vi "Temperature.vi"() -> ()   [LabVIEW 2018, in "Temperature.lvlib"]
uses:
  Temperature.lvlib
  Modbus.xctl
  Sensor.xctl
  Loop Control.xctl
  General Status.xctl
  <vilib>/Platform/TimedLoop/XDataNode/timing_clust.ctl
  <vilib>/Platform/TimedLoop/XDataNode/nitl_modes.ctl
  <vilib>/Platform/TimedLoop/XDataNode/wakeup.ctl
  <vilib>/platform/TimedLoop/XDataNode/XDataNode.xnode
  <vilib>/Platform/TimedLoop/XDataNode/XDNodeRunTimeDep.lvlib
panel:
  out "General Status":u16(xcontrol)
  in  "Loop Control":T1(xcontrol)
  out "Second":cluster{"Value":sgl, "Medium":sgl, "Status":u16}(xcontrol)
  out "Main":cluster{"Value":sgl, "Medium":sgl, "Status":u16}(xcontrol)
  in  "Modbus":T2(xcontrol)
  out "Chart":sgl[](graph)
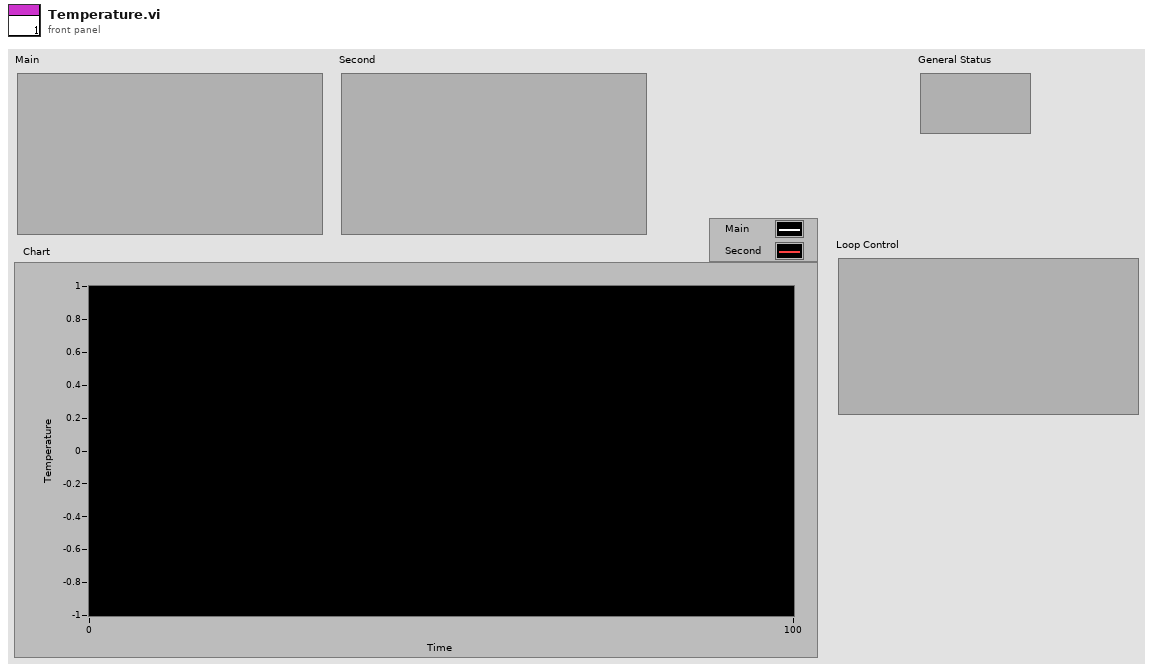
[diagram p1: front panel]
types:
  T1 = cluster{"dt":i64, "error to show":errorcluster, "Active":bool, "stop":bool}
  T2 = cluster{"Communication Error":bool, "Updating":bool, "Off Hook":bool, "Update rate":dbl}
  T3 = typedef "XDNodeRunTimeDep.lvlib/timing_clust.ctl" = cluster{"Expected End [f-1]":u64, "Actual End [f-1]":u64, "Finished Late? [f-1]":bool, "Expected End [i-1]":u64, "Actual End [i-1]":u64, "Finished Late? [i-1]":bool, "Expected Start [i]":u64, "Actual Start [i]":u64, "Expected Start [f]":u64, "Actual Start [f]":u64, "Source Name":string, "Structure Name":string, "Period":i64, "Deadline":i64, "Offset":i64, "Start":i64, "Priority":i32, "Timeout":i32, "Mode":T4, "Wakeup Reason":T5, "Error":errorcluster, "Source Type":string, "Secondary Source Type":string, "Global End Time":u64, "Global Start Time":u64, "Frame Duration":u64, "Iteration Duration":u64, "Assigned CPU":i32, "I/O Scan Engine Mode":u32}
  T4 = typedef "XDNodeRunTimeDep.lvlib/nitl_modes.ctl" = enum32{"No Change", "Process missed periods, maintain original phase", "Discard missed periods, maintain original phase", "Process missed periods, ignore original phase", "Discard missed periods, ignore original phase"}
  T5 = typedef "XDNodeRunTimeDep.lvlib/wakeup.ctl" = enum32{"Normal", "Aborted", "Asynchronous wakeup", "Timing source error", "Timed loop error", "Timeout"}
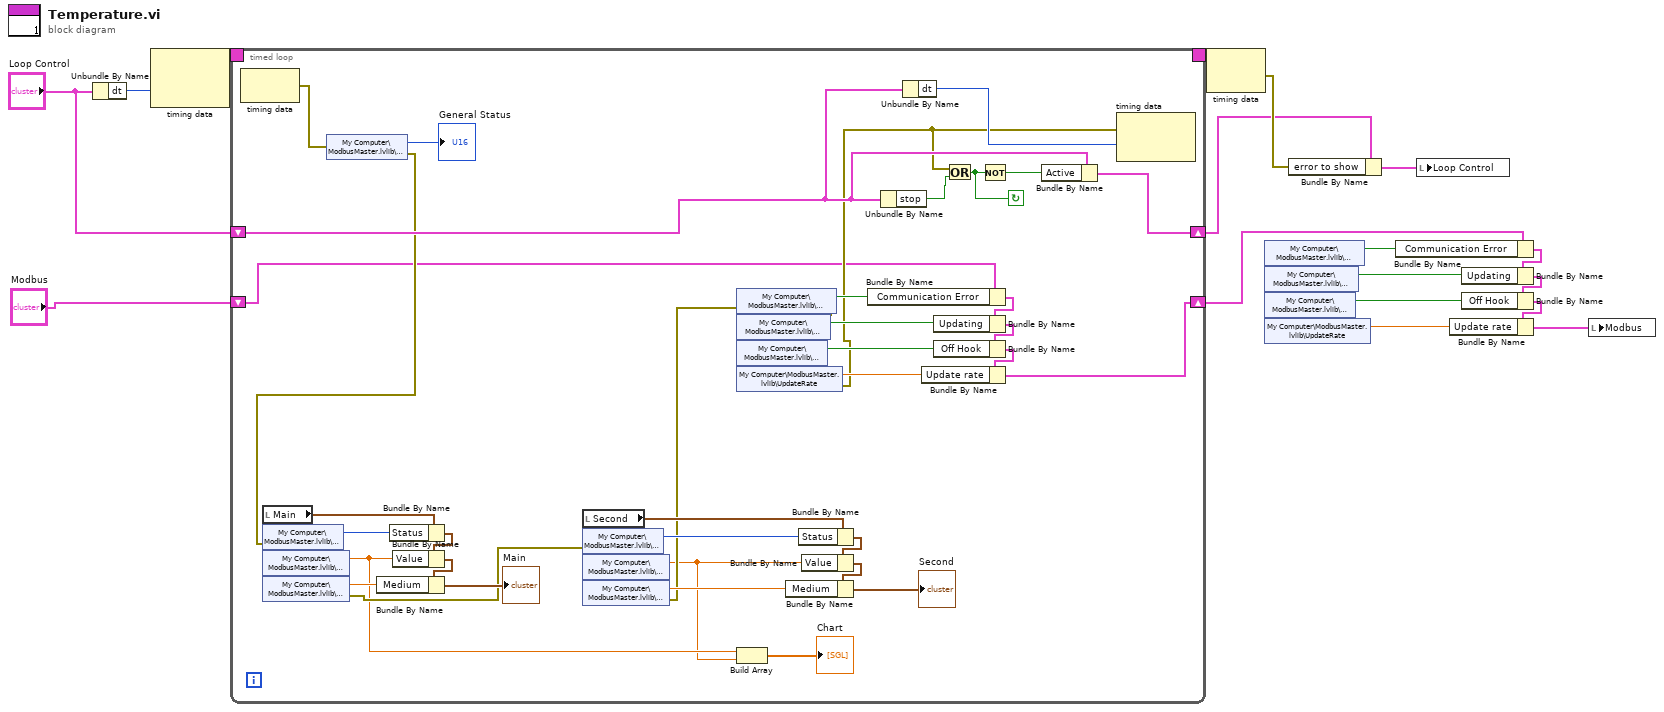
[diagram p0: block diagram]
diagram:
  n1 = Unbundle By Name("Loop Control") -> ("dt"=w15:i64)
  n2 = node-c288(w15) -> (w17:T3)  [unwired: 1 in]
  n3 = timed-loop {
    timing: w17 -> [_]
    timing-out: [_] -> w16
    shift-right: [w54] -> w2
    shift-left: "Loop Control" -> [w55]
    shift-right: [w18] -> w7
    shift-left: "Modbus" -> [w19]
    stop <- w20 continue-if-true
    n4 = node-c288() -> (w36:errorcluster)  [unwired: 1 in]
    n5 = local read "Main"() -> (w50:cluster{"Value":sgl, "Medium":sgl, "Status":u16})
    n6 = shared-variable "My Computer\\ModbusMaster.lvlib\\300001"(error in=w36) -> (→"General Status":u16, error out=w35:errorcluster)
    n7 = shared-variable "My Computer\\ModbusMaster.lvlib\\300005"(error in=w35) -> (w52:u16, error out=w34:errorcluster)
    n8 = shared-variable "My Computer\\ModbusMaster.lvlib\\F300006"(error in=w34) -> (w25:sgl, error out=w33:errorcluster)
    n9 = shared-variable "My Computer\\ModbusMaster.lvlib\\F300008"(error in=w33) -> (w51:sgl, error out=w32:errorcluster)
    n10 = Bundle By Name(cluster=w50, "Status"=w52) -> (w49:cluster{"Value":sgl, "Medium":sgl, "Status":u16})
    n11 = Bundle By Name(cluster=w49, "Value"=w25) -> (w48:cluster{"Value":sgl, "Medium":sgl, "Status":u16})
    n12 = Bundle By Name(cluster=w48, "Medium"=w51) -> (→"Main":cluster{"Value":sgl, "Medium":sgl, "Status":u16})
    n13 = local read "Second"() -> (w44:cluster{"Value":sgl, "Medium":sgl, "Status":u16})
    n14 = shared-variable "My Computer\\ModbusMaster.lvlib\\300010"(error in=w32) -> (w46:u16, error out=w31:errorcluster)
    n15 = shared-variable "My Computer\\ModbusMaster.lvlib\\F300011"(error in=w31) -> (w24:sgl, error out=w30:errorcluster)
    n16 = shared-variable "My Computer\\ModbusMaster.lvlib\\F300013"(error in=w30) -> (w45:sgl, error out=w29:errorcluster)
    n17 = shared-variable "My Computer\\ModbusMaster.lvlib\\CommFail"(error in=w29) -> (w58:bool, error out=w28:errorcluster)
    n18 = shared-variable "My Computer\\ModbusMaster.lvlib\\Updating"(error in=w28) -> (w57:bool, error out=w27:errorcluster)
    n19 = shared-variable "My Computer\\ModbusMaster.lvlib\\OffHook"(error in=w27) -> (w56:bool, error out=w26:errorcluster)
    n20 = shared-variable "My Computer\\ModbusMaster.lvlib\\UpdateRate"(error in=w26) -> (w40:dbl, error out=w22:errorcluster)
    n21 = Build Array(w25, w24) -> (→"Chart":sgl[])
    n22 = Bundle By Name(cluster=w44, "Status"=w46) -> (w43:cluster{"Value":sgl, "Medium":sgl, "Status":u16})
    n23 = Bundle By Name(cluster=w43, "Value"=w24) -> (w42:cluster{"Value":sgl, "Medium":sgl, "Status":u16})
    n24 = Bundle By Name(cluster=w42, "Medium"=w45) -> (→"Second":cluster{"Value":sgl, "Medium":sgl, "Status":u16})
    n25 = Bundle By Name(cluster=w19, "Communication Error"=w58) -> (w39:T2)
    n26 = Unbundle By Name(w55) -> ("stop"=w21:bool)
    n27 = Unbundle By Name(w55) -> ("dt"=w60:i64)
    n28 = Bundle By Name(cluster=w39, "Updating"=w57) -> (w38:T2)
    n29 = Bundle By Name(cluster=w38, "Off Hook"=w56) -> (w37:T2)
    n30 = Bundle By Name(cluster=w37, "Update rate"=w40) -> (w18:T2)
    n31 = Or(x=w22, y=w21) -> (x .or. y?=w20:bool)
    n32 = Not(x=w20) -> (.not. x?=w53:bool)
    n33 = Bundle By Name(cluster=w55, "Active"=w53) -> (w54:T1)
    n34 = node-c288(w22, w60) -> ()  [unwired: 1 out]
  }
  n35 = node-c288(w16) -> (w3:errorcluster)
  n36 = shared-variable "My Computer\\ModbusMaster.lvlib\\CommFail"() -> (w12:bool)  [unwired: 1 in, 1 out]
  n37 = shared-variable "My Computer\\ModbusMaster.lvlib\\Updating"() -> (w11:bool)  [unwired: 1 in, 1 out]
  n38 = shared-variable "My Computer\\ModbusMaster.lvlib\\OffHook"() -> (w10:bool)  [unwired: 1 in, 1 out]
  n39 = shared-variable "My Computer\\ModbusMaster.lvlib\\UpdateRate"() -> (w9:dbl)  [unwired: 1 in, 1 out]
  n40 = Bundle By Name(cluster=w2, "error to show"=w3) -> (w13:T1)
  n41 = Bundle By Name(cluster=w7, "Communication Error"=w12) -> (w6:T2)
  n42 = local write "Loop Control"(w13) -> ()
  n43 = Bundle By Name(cluster=w6, "Updating"=w11) -> (w5:T2)
  n44 = Bundle By Name(cluster=w5, "Off Hook"=w10) -> (w4:T2)
  n45 = Bundle By Name(cluster=w4, "Update rate"=w9) -> (w1:T2)
  n46 = local write "Modbus"(w1) -> ()
